vi "Teardown.vi"(11 "jettl Queue Actor in":refnum<class "jettl Queue Actor.lvclass">) -> (3 "jettl Queue Actor out":refnum<class "jettl Queue Actor.lvclass">)   [LabVIEW 2021, in "jettl.lvlib" / "jettl Queue Actor.lvlib" / "jettl Queue Actor.lvclass"]
uses:
  jettl Queue Actor.lvclass
  State/Teardown State/Teardown State.lvclass
  jettl.lvlib
  C:/git/jettl/src/Actor/Queue Actor/Queue Actor.lvclass
  C:/git/jettl/src/Actor/Actor/Actor.lvclass
  C:/git/jettl/src/Actor/Msgs/Create/Create/Create.lvclass
  C:/git/jettl/src/Actor/Msgs/Event Create/Event Create/Event Create.lvclass
  C:/git/jettl/src/Actor/Msgs/Event Last Ack/Event Last Ack/Event Last Ack.lvclass
  C:/git/jettl/src/Actor/Msgs/Event Teardown/Event Teardown/Event Teardown.lvclass
  C:/git/jettl/src/Actor/Msgs/Last Ack/Last Ack/Last Ack.lvclass
  C:/git/jettl/src/Actor/Msgs/Setup/Setup/Setup.lvclass
  C:/git/jettl/src/Actor/Msgs/Teardown/Teardown/Teardown.lvclass
  C:/git/jettl/src/jettl/jettl Queue Actor/jettl Queue Actor/jettl Queue Actor.lvclass
  C:/git/jettl/src/jettl/jettl Queue Actor/State/Teardown State/Teardown State.lvclass
  C:/git/jettl/src/jettl/jettl Queue Actor/State/State/State.lvclass
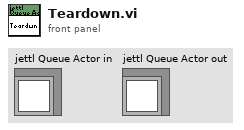
[diagram p1: front panel]
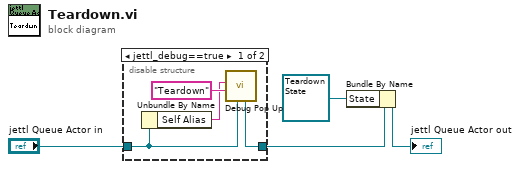
[diagram p0: block diagram]
diagram:
  n1 = disable-structure shown="jettl_debug==true" {
    disable-tunnel: "jettl Queue Actor in" -> [w6 _]
    disable-tunnel: [w7 _] -> w1
    frame condition #0 (active) {
      n2 = Unbundle By Name(w6) -> ("Self Alias"=w5:string)
      n3 = call "Debug Pop Up.vi"("Input"=w6, "Method"="Teardown", "Alias"=w5) -> ("Output"=w7:refnum<class "jettl Queue Actor.lvclass">)  [unwired: 8 in]
    }
    frame condition #1 {
    }
  }
  n4 = Bundle By Name(cluster=w1, "State"=refnum<class "Teardown State.lvclass"> refnum ("LVCAM.lvlib:Destroying Self Actor State.lvclass")) -> (→"jettl Queue Actor out":refnum<class "jettl Queue Actor.lvclass">)
